vi "数据处理整合 (子VI).vi"(11 "枚举":enum16{"实时数据排序", "小时数据排序"}(ring)) -> (3 "已排序的数组":string[](array[string]))   [LabVIEW 2016, in "数据传输系统-02.lvlib"]
uses:
  <userlib>/_OpenG.lib/array/array.llb/Remove Duplicates from 1D Array (String)__ogtk.vi
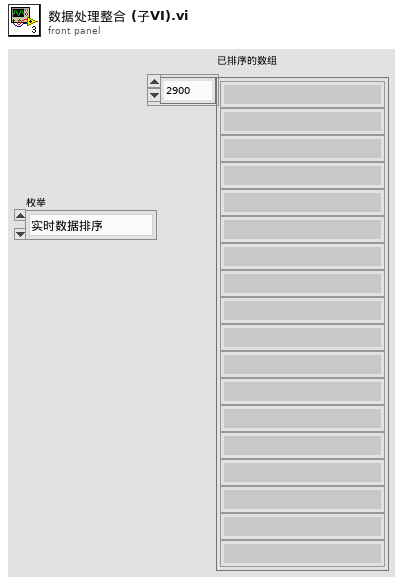
[diagram p1: front panel]
types:
  T1 = cluster{"PH":string[][], "CODCr":string[][], "氨氮":string[][], "CODMn":string[][], "总氮":string[][], "总磷":string[][], "电导率":string[][], "水温":string[][], "DO":string[][], "浊度":string[][], "叶绿素":string[][], "藻密度":string[][], "铜":string[][], "盐度":string[][], "水位":string[][], "流速":string[][], "瞬时流量":string[][], "累积流量":string[][], "亚硝酸盐":string[][], "硫化物":string[][], "ORP":string[][], "铅":string[][], "镉":string[][], "锌":string[][], "镍":string[][], "锰":string[][], "汞":string[][], "气温":string[][], "气压":string[][], "风速":string[][], "风向":string[][], "盐度 2":string[][], "磷酸盐":string[][], "硝氮":string[][], "氟化物":string[][]}
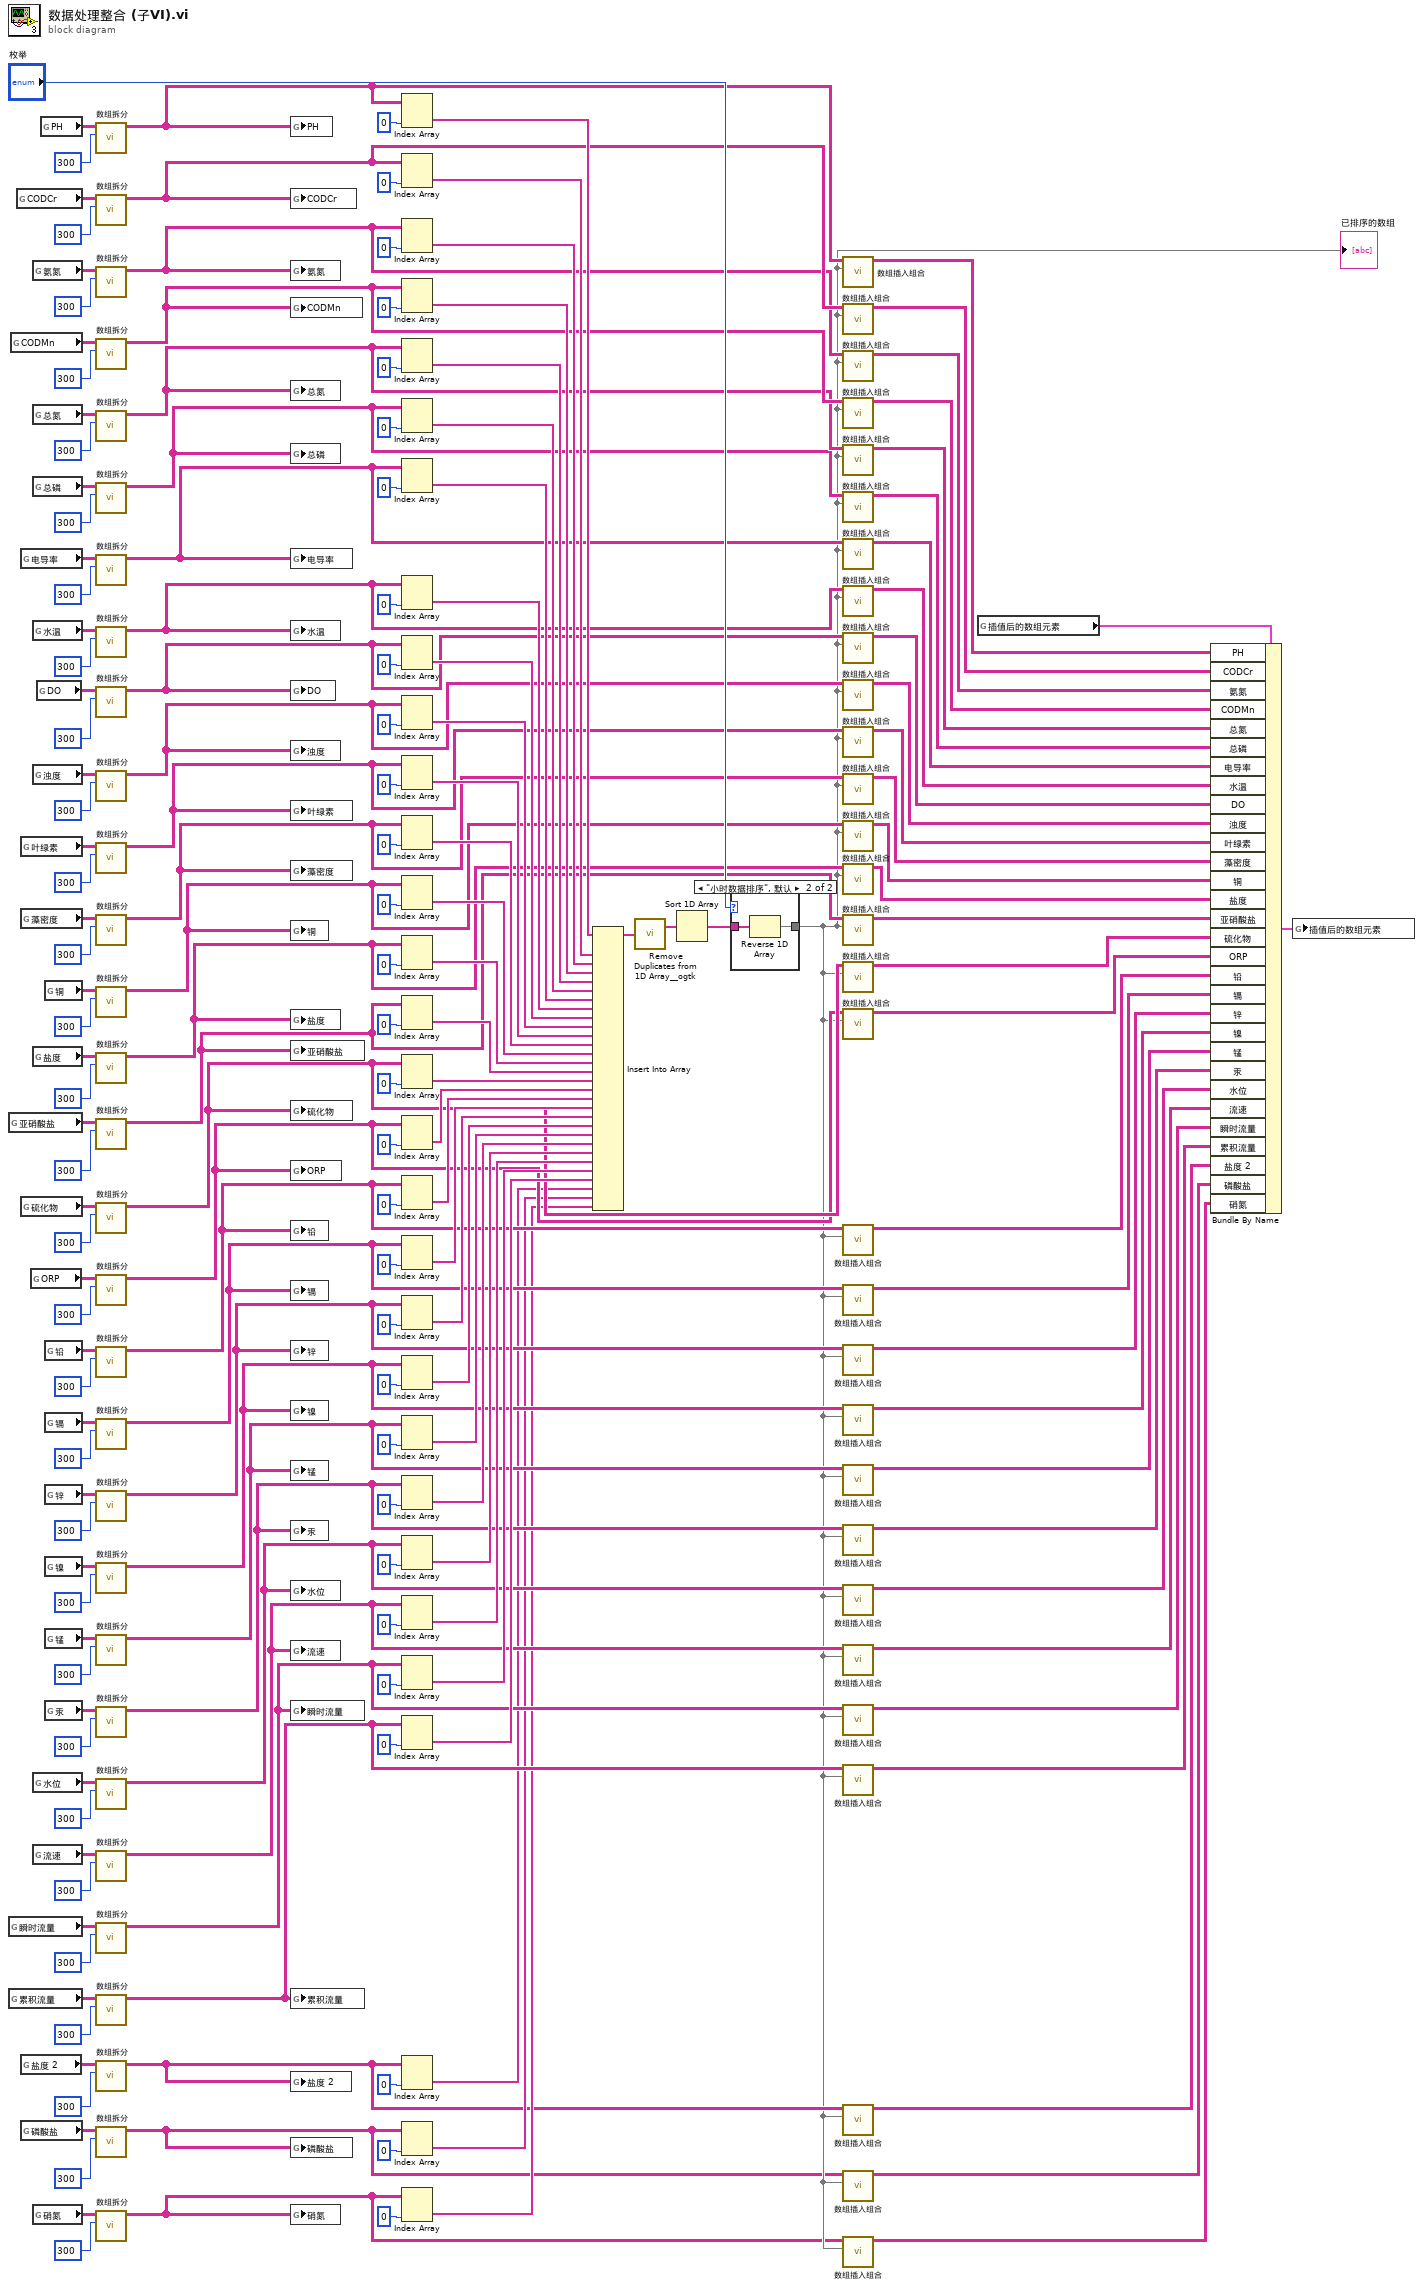
[diagram p0: block diagram]
diagram:
  n1 = global read "全局 所有参数.vi" "亚硝酸盐"() -> (w51:string[][])
  n2 = global read "全局 所有参数.vi" "瞬时流量"() -> (w27:string[][])
  n3 = global read "全局 所有参数.vi" "累积流量"() -> (w26:string[][])
  n4 = global read "全局 所有参数.vi" "CODMn"() -> (w90:string[][])
  n5 = global read "全局 所有参数.vi" "CODCr"() -> (w96:string[][])
  n6 = global read "全局 所有参数.vi" "电导率"() -> (w80:string[][])
  n7 = global read "全局 所有参数.vi" "叶绿素"() -> (w67:string[][])
  n8 = global read "全局 所有参数.vi" "藻密度"() -> (w66:string[][])
  n9 = global read "全局 所有参数.vi" "硫化物"() -> (w50:string[][])
  n10 = global read "全局 所有参数.vi" "盐度 2"() -> (w13:string[][])
  n11 = global read "全局 所有参数.vi" "磷酸盐"() -> (w12:string[][])
  n12 = global read "全局 所有参数.vi" "ORP"() -> (w49:string[][])
  n13 = global read "全局 所有参数.vi" "氨氮"() -> (w93:string[][])
  n14 = global read "全局 所有参数.vi" "总氮"() -> (w87:string[][])
  n15 = global read "全局 所有参数.vi" "总磷"() -> (w81:string[][])
  n16 = global read "全局 所有参数.vi" "水温"() -> (w79:string[][])
  n17 = global read "全局 所有参数.vi" "浊度"() -> (w68:string[][])
  n18 = global read "全局 所有参数.vi" "盐度"() -> (w64:string[][])
  n19 = global read "全局 所有参数.vi" "水位"() -> (w29:string[][])
  n20 = global read "全局 所有参数.vi" "流速"() -> (w28:string[][])
  n21 = global read "全局 所有参数.vi" "硝氮"() -> (w11:string[][])
  n22 = global read "全局 所有参数.vi" "DO"() -> (w78:string[][])
  n23 = global read "全局 所有参数.vi" "PH"() -> (w99:string[][])
  n24 = global read "全局 所有参数.vi" "铜"() -> (w65:string[][])
  n25 = global read "全局 所有参数.vi" "铅"() -> (w48:string[][])
  n26 = global read "全局 所有参数.vi" "镉"() -> (w47:string[][])
  n27 = global read "全局 所有参数.vi" "锌"() -> (w46:string[][])
  n28 = global read "全局 所有参数.vi" "镍"() -> (w45:string[][])
  n29 = global read "全局 所有参数.vi" "锰"() -> (w31:string[][])
  n30 = global read "全局 所有参数.vi" "汞"() -> (w30:string[][])
  n31 = call "数组拆分.vi"("拆分大小"=300, "输入数据"=w99) -> ("输出数组"=w98:string[][])  [unwired: 8 in, 1 out]
  n32 = call "数组拆分.vi"("拆分大小"=300, "输入数据"=w96) -> ("输出数组"=w95:string[][])  [unwired: 8 in, 1 out]
  n33 = call "数组拆分.vi"("拆分大小"=300, "输入数据"=w93) -> ("输出数组"=w92:string[][])  [unwired: 8 in, 1 out]
  n34 = call "数组拆分.vi"("拆分大小"=300, "输入数据"=w90) -> ("输出数组"=w89:string[][])  [unwired: 8 in, 1 out]
  n35 = call "数组拆分.vi"("拆分大小"=300, "输入数据"=w87) -> ("输出数组"=w86:string[][])  [unwired: 8 in, 1 out]
  n36 = call "数组拆分.vi"("拆分大小"=300, "输入数据"=w81) -> ("输出数组"=w74:string[][])  [unwired: 8 in, 1 out]
  n37 = call "数组拆分.vi"("拆分大小"=300, "输入数据"=w80) -> ("输出数组"=w75:string[][])  [unwired: 8 in, 1 out]
  n38 = call "数组拆分.vi"("拆分大小"=300, "输入数据"=w79) -> ("输出数组"=w76:string[][])  [unwired: 8 in, 1 out]
  n39 = call "数组拆分.vi"("拆分大小"=300, "输入数据"=w78) -> ("输出数组"=w77:string[][])  [unwired: 8 in, 1 out]
  n40 = call "数组拆分.vi"("拆分大小"=300, "输入数据"=w68) -> ("输出数组"=w63:string[][])  [unwired: 8 in, 1 out]
  n41 = call "数组拆分.vi"("拆分大小"=300, "输入数据"=w67) -> ("输出数组"=w59:string[][])  [unwired: 8 in, 1 out]
  n42 = call "数组拆分.vi"("拆分大小"=300, "输入数据"=w66) -> ("输出数组"=w60:string[][])  [unwired: 8 in, 1 out]
  n43 = call "数组拆分.vi"("拆分大小"=300, "输入数据"=w65) -> ("输出数组"=w61:string[][])  [unwired: 8 in, 1 out]
  n44 = call "数组拆分.vi"("拆分大小"=300, "输入数据"=w64) -> ("输出数组"=w62:string[][])  [unwired: 8 in, 1 out]
  n45 = call "数组拆分.vi"("拆分大小"=300, "输入数据"=w51) -> ("输出数组"=w44:string[][])  [unwired: 8 in, 1 out]
  n46 = call "数组拆分.vi"("拆分大小"=300, "输入数据"=w50) -> ("输出数组"=w43:string[][])  [unwired: 8 in, 1 out]
  n47 = call "数组拆分.vi"("拆分大小"=300, "输入数据"=w49) -> ("输出数组"=w42:string[][])  [unwired: 8 in, 1 out]
  n48 = call "数组拆分.vi"("拆分大小"=300, "输入数据"=w48) -> ("输出数组"=w41:string[][])  [unwired: 8 in, 1 out]
  n49 = call "数组拆分.vi"("拆分大小"=300, "输入数据"=w47) -> ("输出数组"=w40:string[][])  [unwired: 8 in, 1 out]
  n50 = call "数组拆分.vi"("拆分大小"=300, "输入数据"=w46) -> ("输出数组"=w39:string[][])  [unwired: 8 in, 1 out]
  n51 = call "数组拆分.vi"("拆分大小"=300, "输入数据"=w45) -> ("输出数组"=w38:string[][])  [unwired: 8 in, 1 out]
  n52 = call "数组拆分.vi"("拆分大小"=300, "输入数据"=w31) -> ("输出数组"=w25:string[][])  [unwired: 8 in, 1 out]
  n53 = call "数组拆分.vi"("拆分大小"=300, "输入数据"=w30) -> ("输出数组"=w23:string[][])  [unwired: 8 in, 1 out]
  n54 = call "数组拆分.vi"("拆分大小"=300, "输入数据"=w29) -> ("输出数组"=w24:string[][])  [unwired: 8 in, 1 out]
  n55 = call "数组拆分.vi"("拆分大小"=300, "输入数据"=w28) -> ("输出数组"=w22:string[][])  [unwired: 8 in, 1 out]
  n56 = call "数组拆分.vi"("拆分大小"=300, "输入数据"=w27) -> ("输出数组"=w21:string[][])  [unwired: 8 in, 1 out]
  n57 = call "数组拆分.vi"("拆分大小"=300, "输入数据"=w26) -> ("输出数组"=w20:string[][])  [unwired: 8 in, 1 out]
  n58 = call "数组拆分.vi"("拆分大小"=300, "输入数据"=w13) -> ("输出数组"=w7:string[][])  [unwired: 8 in, 1 out]
  n59 = call "数组拆分.vi"("拆分大小"=300, "输入数据"=w12) -> ("输出数组"=w5:string[][])  [unwired: 8 in, 1 out]
  n60 = call "数组拆分.vi"("拆分大小"=300, "输入数据"=w11) -> ("输出数组"=w4:string[][])  [unwired: 8 in, 1 out]
  n61 = global write "全局 所有参数.vi" "PH"(w98) -> ()
  n62 = global write "全局 所有参数.vi" "CODCr"(w95) -> ()
  n63 = global write "全局 所有参数.vi" "氨氮"(w92) -> ()
  n64 = global write "全局 所有参数.vi" "CODMn"(w89) -> ()
  n65 = global write "全局 所有参数.vi" "总氮"(w86) -> ()
  n66 = global write "全局 所有参数.vi" "总磷"(w74) -> ()
  n67 = global write "全局 所有参数.vi" "电导率"(w75) -> ()
  n68 = global write "全局 所有参数.vi" "水温"(w76) -> ()
  n69 = global write "全局 所有参数.vi" "DO"(w77) -> ()
  n70 = global write "全局 所有参数.vi" "浊度"(w63) -> ()
  n71 = global write "全局 所有参数.vi" "叶绿素"(w59) -> ()
  n72 = global write "全局 所有参数.vi" "藻密度"(w60) -> ()
  n73 = global write "全局 所有参数.vi" "铜"(w61) -> ()
  n74 = global write "全局 所有参数.vi" "盐度"(w62) -> ()
  n75 = global write "全局 所有参数.vi" "亚硝酸盐"(w44) -> ()
  n76 = global write "全局 所有参数.vi" "硫化物"(w43) -> ()
  n77 = global write "全局 所有参数.vi" "ORP"(w42) -> ()
  n78 = global write "全局 所有参数.vi" "铅"(w41) -> ()
  n79 = global write "全局 所有参数.vi" "镉"(w40) -> ()
  n80 = global write "全局 所有参数.vi" "锌"(w39) -> ()
  n81 = global write "全局 所有参数.vi" "镍"(w38) -> ()
  n82 = global write "全局 所有参数.vi" "锰"(w25) -> ()
  n83 = global write "全局 所有参数.vi" "汞"(w23) -> ()
  n84 = global write "全局 所有参数.vi" "水位"(w24) -> ()
  n85 = global write "全局 所有参数.vi" "流速"(w22) -> ()
  n86 = global write "全局 所有参数.vi" "瞬时流量"(w21) -> ()
  n87 = global write "全局 所有参数.vi" "累积流量"(w20) -> ()
  n88 = global write "全局 所有参数.vi" "盐度 2"(w7) -> ()
  n89 = global write "全局 所有参数.vi" "磷酸盐"(w5) -> ()
  n90 = global write "全局 所有参数.vi" "硝氮"(w4) -> ()
  n91 = Index Array(array=w98, index (col)=0 ("索引 (行)")) -> (element=w163:string[])  [unwired: 1 in]
  n92 = Index Array(array=w95, index (col)=0 ("索引 (行)")) -> (element=w164:string[])  [unwired: 1 in]
  n93 = Index Array(array=w92, index (col)=0 ("索引 (行)")) -> (element=w165:string[])  [unwired: 1 in]
  n94 = Index Array(array=w89, index (col)=0 ("索引 (行)")) -> (element=w166:string[])  [unwired: 1 in]
  n95 = Index Array(array=w86, index (col)=0 ("索引 (行)")) -> (element=w167:string[])  [unwired: 1 in]
  n96 = Index Array(array=w74, index (col)=0 ("索引 (行)")) -> (element=w168:string[])  [unwired: 1 in]
  n97 = Index Array(array=w75, index (col)=0 ("索引 (行)")) -> (element=w169:string[])  [unwired: 1 in]
  n98 = Index Array(array=w76, index (col)=0 ("索引 (行)")) -> (element=w170:string[])  [unwired: 1 in]
  n99 = Index Array(array=w77, index (col)=0 ("索引 (行)")) -> (element=w171:string[])  [unwired: 1 in]
  n100 = Index Array(array=w63, index (col)=0 ("索引 (行)")) -> (element=w172:string[])  [unwired: 1 in]
  n101 = Index Array(array=w59, index (col)=0 ("索引 (行)")) -> (element=w173:string[])  [unwired: 1 in]
  n102 = Index Array(array=w60, index (col)=0 ("索引 (行)")) -> (element=w174:string[])  [unwired: 1 in]
  n103 = Index Array(array=w61, index (col)=0 ("索引 (行)")) -> (element=w147:string[])  [unwired: 1 in]
  n104 = Index Array(array=w62, index (col)=0 ("索引 (行)")) -> (element=w146:string[])  [unwired: 1 in]
  n105 = Index Array(array=w44, index (col)=0 ("索引 (行)")) -> (element=w132:string[])  [unwired: 1 in]
  n106 = Index Array(array=w43, index (col)=0 ("索引 (行)")) -> (element=w133:string[])  [unwired: 1 in]
  n107 = Index Array(array=w42, index (col)=0 ("索引 (行)")) -> (element=w134:string[])  [unwired: 1 in]
  n108 = Index Array(array=w41, index (col)=0 ("索引 (行)")) -> (element=w124:string[])  [unwired: 1 in]
  n109 = Index Array(array=w40, index (col)=0 ("索引 (行)")) -> (element=w123:string[])  [unwired: 1 in]
  n110 = Index Array(array=w39, index (col)=0 ("索引 (行)")) -> (element=w122:string[])  [unwired: 1 in]
  n111 = Index Array(array=w38, index (col)=0 ("索引 (行)")) -> (element=w118:string[])  [unwired: 1 in]
  n112 = Index Array(array=w25, index (col)=0 ("索引 (行)")) -> (element=w117:string[])  [unwired: 1 in]
  n113 = Index Array(array=w23, index (col)=0 ("索引 (行)")) -> (element=w116:string[])  [unwired: 1 in]
  n114 = Index Array(array=w24, index (col)=0 ("索引 (行)")) -> (element=w108:string[])  [unwired: 1 in]
  n115 = Index Array(array=w22, index (col)=0 ("索引 (行)")) -> (element=w107:string[])  [unwired: 1 in]
  n116 = Index Array(array=w21, index (col)=0 ("索引 (行)")) -> (element=w106:string[])  [unwired: 1 in]
  n117 = Index Array(array=w20, index (col)=0 ("索引 (行)")) -> (element=w105:string[])  [unwired: 1 in]
  n118 = Index Array(array=w7, index (col)=0 ("索引 (行)")) -> (element=w10:string[])  [unwired: 1 in]
  n119 = Index Array(array=w5, index (col)=0 ("索引 (行)")) -> (element=w9:string[])  [unwired: 1 in]
  n120 = Index Array(array=w4, index (col)=0 ("索引 (行)")) -> (element=w8:string[])  [unwired: 1 in]
  n121 = Insert Into Array(array=w163, new element #1=w164, new element #2=w165, new element #3=w166, new element #4=w167, new element #5=w168, new element #6=w169, new element #7=w170, new element #8=w171, new element #9=w172, new element #10=w173, new element #11=w174, new element #12=w147, new element #13=w146, new element #14=w132, new element #15=w133, new element #16=w134, new element #17=w124, new element #18=w123, new element #19=w122, new element #20=w118, new element #21=w117, new element #22=w116, new element #23=w108, new element #24=w107, new element #25=w106, new element #26=w105, new element #27=w10, new element #28=w9, new element #29=w8) -> (w175:string[])  [unwired: 1 in]
  n122 = call-poly <userlib>:"Remove Duplicates from 1D Array__ogtk.vi"("Input Array"=w175) -> ("Output Array"=w162:string[])  [unwired: 1 out]
  n123 = Sort 1D Array(array=w162) -> (sorted array=w148:string[])
  n124 = case shown="\"小时数据排序\", 默认" "枚举" {
    tunnel: w148 -> [w188 w190]
    tunnel: [w188 w189] -> w6
    frame "实时数据排序" {
    }
    frame "小时数据排序", Default {
      n125 = Reverse 1D Array(array=w190) -> (reversed array=w189:string[])
    }
  }
  "已排序的数组" <- w6
  n126 = call "数组插入组合.vi"("排序后的一维数组"=w6, "输入数组"=w98) -> ("输出结果"=w176:string[][])  [unwired: 9 in]
  n127 = call "数组插入组合.vi"("排序后的一维数组"=w6, "输入数组"=w95) -> ("输出结果"=w177:string[][])  [unwired: 9 in]
  n128 = call "数组插入组合.vi"("排序后的一维数组"=w6, "输入数组"=w92) -> ("输出结果"=w178:string[][])  [unwired: 9 in]
  n129 = call "数组插入组合.vi"("排序后的一维数组"=w6, "输入数组"=w89) -> ("输出结果"=w179:string[][])  [unwired: 9 in]
  n130 = call "数组插入组合.vi"("排序后的一维数组"=w6, "输入数组"=w86) -> ("输出结果"=w180:string[][])  [unwired: 9 in]
  n131 = call "数组插入组合.vi"("排序后的一维数组"=w6, "输入数组"=w74) -> ("输出结果"=w181:string[][])  [unwired: 9 in]
  n132 = call "数组插入组合.vi"("排序后的一维数组"=w6, "输入数组"=w75) -> ("输出结果"=w182:string[][])  [unwired: 9 in]
  n133 = call "数组插入组合.vi"("排序后的一维数组"=w6, "输入数组"=w76) -> ("输出结果"=w183:string[][])  [unwired: 9 in]
  n134 = call "数组插入组合.vi"("排序后的一维数组"=w6, "输入数组"=w77) -> ("输出结果"=w184:string[][])  [unwired: 9 in]
  n135 = call "数组插入组合.vi"("排序后的一维数组"=w6, "输入数组"=w63) -> ("输出结果"=w185:string[][])  [unwired: 9 in]
  n136 = call "数组插入组合.vi"("排序后的一维数组"=w6, "输入数组"=w59) -> ("输出结果"=w186:string[][])  [unwired: 9 in]
  n137 = call "数组插入组合.vi"("排序后的一维数组"=w6, "输入数组"=w60) -> ("输出结果"=w187:string[][])  [unwired: 9 in]
  n138 = call "数组插入组合.vi"("排序后的一维数组"=w6, "输入数组"=w61) -> ("输出结果"=w145:string[][])  [unwired: 9 in]
  n139 = call "数组插入组合.vi"("排序后的一维数组"=w6, "输入数组"=w62) -> ("输出结果"=w144:string[][])  [unwired: 9 in]
  n140 = call "数组插入组合.vi"("排序后的一维数组"=w6, "输入数组"=w44) -> ("输出结果"=w137:string[][])  [unwired: 9 in]
  n141 = call "数组插入组合.vi"("排序后的一维数组"=w6, "输入数组"=w43) -> ("输出结果"=w135:string[][])  [unwired: 9 in]
  n142 = call "数组插入组合.vi"("排序后的一维数组"=w6, "输入数组"=w42) -> ("输出结果"=w136:string[][])  [unwired: 9 in]
  n143 = call "数组插入组合.vi"("排序后的一维数组"=w6, "输入数组"=w41) -> ("输出结果"=w127:string[][])  [unwired: 9 in]
  n144 = call "数组插入组合.vi"("排序后的一维数组"=w6, "输入数组"=w40) -> ("输出结果"=w126:string[][])  [unwired: 9 in]
  n145 = call "数组插入组合.vi"("排序后的一维数组"=w6, "输入数组"=w39) -> ("输出结果"=w125:string[][])  [unwired: 9 in]
  n146 = call "数组插入组合.vi"("排序后的一维数组"=w6, "输入数组"=w38) -> ("输出结果"=w115:string[][])  [unwired: 9 in]
  n147 = call "数组插入组合.vi"("排序后的一维数组"=w6, "输入数组"=w25) -> ("输出结果"=w114:string[][])  [unwired: 9 in]
  n148 = call "数组插入组合.vi"("排序后的一维数组"=w6, "输入数组"=w23) -> ("输出结果"=w113:string[][])  [unwired: 9 in]
  n149 = call "数组插入组合.vi"("排序后的一维数组"=w6, "输入数组"=w24) -> ("输出结果"=w104:string[][])  [unwired: 9 in]
  n150 = call "数组插入组合.vi"("排序后的一维数组"=w6, "输入数组"=w22) -> ("输出结果"=w103:string[][])  [unwired: 9 in]
  n151 = call "数组插入组合.vi"("排序后的一维数组"=w6, "输入数组"=w21) -> ("输出结果"=w102:string[][])  [unwired: 9 in]
  n152 = call "数组插入组合.vi"("排序后的一维数组"=w6, "输入数组"=w20) -> ("输出结果"=w101:string[][])  [unwired: 9 in]
  n153 = call "数组插入组合.vi"("排序后的一维数组"=w6, "输入数组"=w7) -> ("输出结果"=w3:string[][])  [unwired: 9 in]
  n154 = call "数组插入组合.vi"("排序后的一维数组"=w6, "输入数组"=w5) -> ("输出结果"=w2:string[][])  [unwired: 9 in]
  n155 = call "数组插入组合.vi"("排序后的一维数组"=w6, "输入数组"=w4) -> ("输出结果"=w1:string[][])  [unwired: 9 in]
  n156 = global read "插值后的新数组.vi" "插值后的数组元素"() -> (w141:T1)
  n157 = Bundle By Name(cluster=w141, "PH"=w176, "CODCr"=w177, "氨氮"=w178, "CODMn"=w179, "总氮"=w180, "总磷"=w181, "电导率"=w182, "水温"=w183, "DO"=w184, "浊度"=w185, "叶绿素"=w186, "藻密度"=w187, "铜"=w145, "盐度"=w144, "亚硝酸盐"=w137, "硫化物"=w135, "ORP"=w136, "铅"=w127, "镉"=w126, "锌"=w125, "镍"=w115, "锰"=w114, "汞"=w113, "水位"=w104, "流速"=w103, "瞬时流量"=w102, "累积流量"=w101, "盐度 2"=w3, "磷酸盐"=w2, "硝氮"=w1) -> (w131:T1)
  n158 = global write "插值后的新数组.vi" "插值后的数组元素"(w131) -> ()
